vi "Clear Obstructing Path.vi"(8 "error in":errorcluster, 11 "2525 in":refnum<class "2525.lvclass">) -> (0 "error out":errorcluster, 3 "2525 out":refnum<class "2525.lvclass">)   [LabVIEW 2019, in "2525.lvlib" / "2525.lvclass"]
uses:
  Library/2525.lvclass
  Library/2525.lvclass/2525.ctl
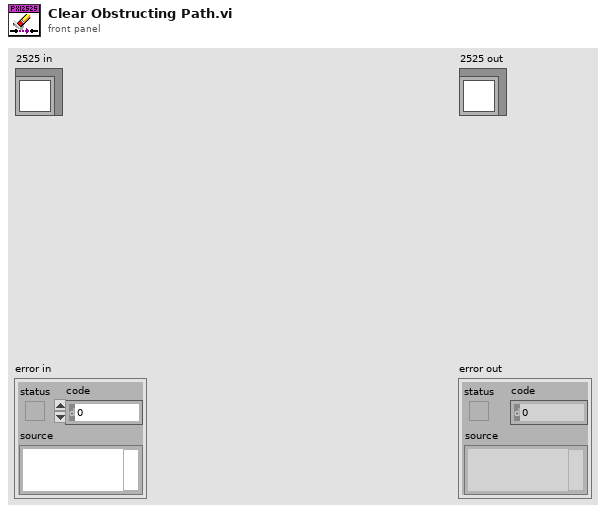
[diagram p1: front panel]
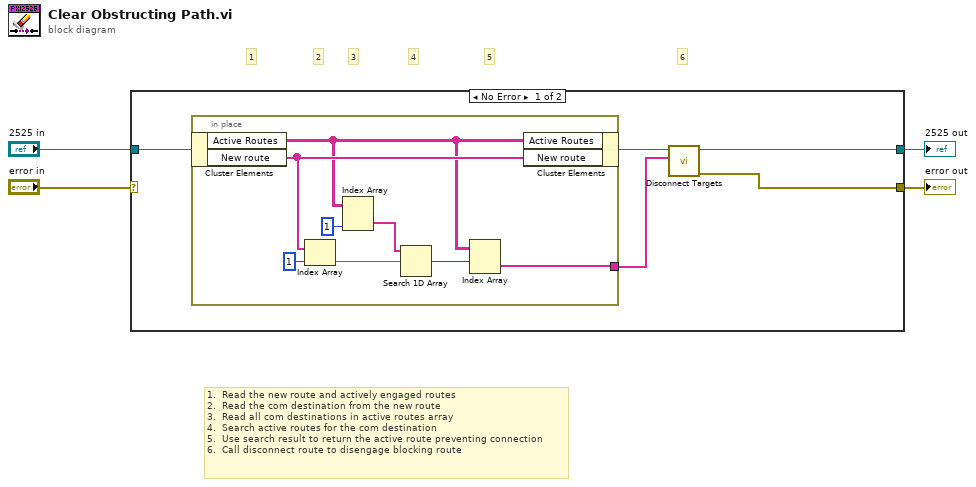
[diagram p0: block diagram]
diagram:
  # "1.  Read the new route and actively engaged routes\n2.  Read the com destination from the new route\n3.  Read all com destinations in active routes array\n4.  Search active routes for the com destination\n5.  Use search result to return the active route preventing connection\n6.  Call disconnect route to disengage blocking route"
  # "6"
  # "5"
  # "4"
  # "3"
  # "2"
  # "1"
  n1 = case shown="No Error" "error in" {
    selector: "error in" -> [_ w19]
    tunnel: [w5 w19] -> w3
    tunnel: [w6 w18] -> w1
    tunnel: "2525 in" -> [w9 w18]
    frame No Error {
      n2 = in-place {
        in-place-border: [w10] -> w8
        n3 = in-place-cluster #1(w9) -> ("Active Routes"=w11:string[][], "New route"=w17:string[])
        n4 = Index Array(array=w17, index=1) -> (element=w15:string)
        n5 = Index Array(array=w11, index (col)=1 ("disabled index (col)")) -> (element=w16:string[])  [unwired: 1 in]
        n6 = Search 1D Array(1D array=w16, element=w15) -> (index of element=w12:i32)  [unwired: 1 in]
        n7 = Index Array(array=w11, index (row)=w12) -> (element=w10:string[])  [unwired: 1 in]
        n8 = in-place-cluster #1("Active Routes"=w11, "New route"=w17) -> (w7:refnum<class "2525.lvclass">)
      }
      n9 = call "Disconnect Targets.vi"("Disconnect targets"=w8, "2525 in"=w7) -> ("error out"=w5:errorcluster, "2525 out"=w6:refnum<class "2525.lvclass">)  [unwired: 8 in]
    }
    frame Error {
    }
  }
  "error out" <- w3
  "2525 out" <- w1
